vi "Interpret Set-Point Driver Message.vi"() -> (0 "Pause":bool)   [LabVIEW 2013]
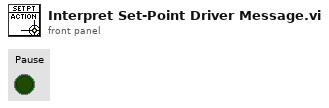
[diagram p1: front panel]
types:
  T1 = typedef "Set-Point Driver Messages.ctl" = enum16{"Begin Enforcement", "Cease Enforcement"}
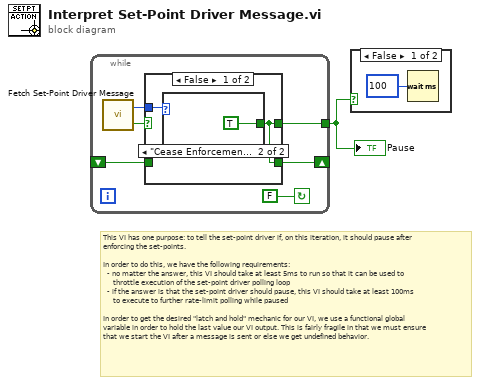
[diagram p0: block diagram]
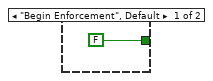
[diagram p3: hidden frame]
diagram:
  # "This VI has one purpose: to tell the set-point driver if, on this iteration, it should pause after\nenforcing the set-points. \n\nIn order to do this, we have the following requirements:\n  - no matter the answer, this VI should take at least 5ms to run so that it can be used to\n     throttle execution of the set-point driver polling loop\n  - if the answer is that the set-point driver should pause, this VI should take at least 100ms\n     to execute to further rate-limit polling while paused\n\nIn order to get the desired \"latch and hold\" mechanic for our VI, we use a functional global\nvariable in order to hold the last value our VI output. This is fairly fragile in that we must ensure\nthat we start the VI after a message is sent or else we get undefined behavior."
  n1 = while {
    shift-right: [w4] -> _
    shift-left: _ -> [w3]
    tunnel: [w2] -> w1
    stop <- FALSE continue-if-true
    n2 = call "Fetch Set-Point Driver Message.vi"() -> ("Timed Out"=w5:bool, "Message"=w6:T1)  [unwired: 2 in]
    n3 = case shown="False" w5 {
      tunnel: w6 -> [w9 _]
      tunnel: [w8 w12] -> w2
      tunnel: [w8 w12] -> w4
      tunnel: w3 -> [_ w12]
      frame False {
        n4 = case shown="\"Cease Enforcement\"" w9 {
          tunnel: [FALSE TRUE] -> w8
          frame "Begin Enforcement", Default {
          }
          frame "Cease Enforcement" {
          }
        }
      }
      frame True {
      }
    }
  }
  "Pause" <- w1
  n5 = case shown="False" w1 {
    frame False {
      n6 = Wait (ms)(milliseconds to wait=u32 100) -> ()  [unwired: 1 out]
    }
    frame True {
    }
  }
